vi "Elemente auswerten_Debug_Ablaufvariant.vi"(0 "GObject (Eingang)":refnum<vi>, 3 "Sprachauswahl":u16, 5 "Fehler (Eingang, kein Fehler)":errorcluster, 6 "Index":i32, 8 "ClassID":u32) -> (14 "Strings [4]":string[](array[string]), 15 "Cluster Elemente[]":refnum<vi>[](array[refnum]), 19 "error out":errorcluster)   [LabVIEW 2020, in "Sprachverwaltung.lvlib"]
uses:
  Sprachverwaltung.lvlib
  FGV Aktion Tabelle zerlegen.ctl
panel:
  # "3 Generic \n4 Decoration \n5 Text \n6 Control \n7 ColorBox \n8 Boolean \n9 RefNum \n10 Variant \n11 Path \n12 ListBox \n13 Table \n14 Array \n15 Picture \n16 ActiveXContainer \n17 Numeric \n18 Digital \n19 NamedNumeric \n20 ColorRamp \n21 Slide \n22 GraphOrChart \n23 WaveformChart \n24 WaveformGraph \n25 IntensityChart \n26 IntensityGraph \n27 String \n28 IOName \n29 ComboBox \n30 Cluster \n31 Panel \n32 Knob \n33 NumWithScale \n34 Ring \n35 Enum \n36 GObject \n37 Plot \n38 Cursor \n39 NumericText \n40 Scale \n41 ColorScale \n42 GraphScale \n43 ColorGraphScale \n44 TypedRefNum \n45 OldKnobScale \n46 MCListbox \n47 MeasureData \n48 BVTag \n49 DAQName \n50 VISAName \n51 IVIName \n52 SlideScale \n54 Page \n55 TabControl \n56 ConPane"
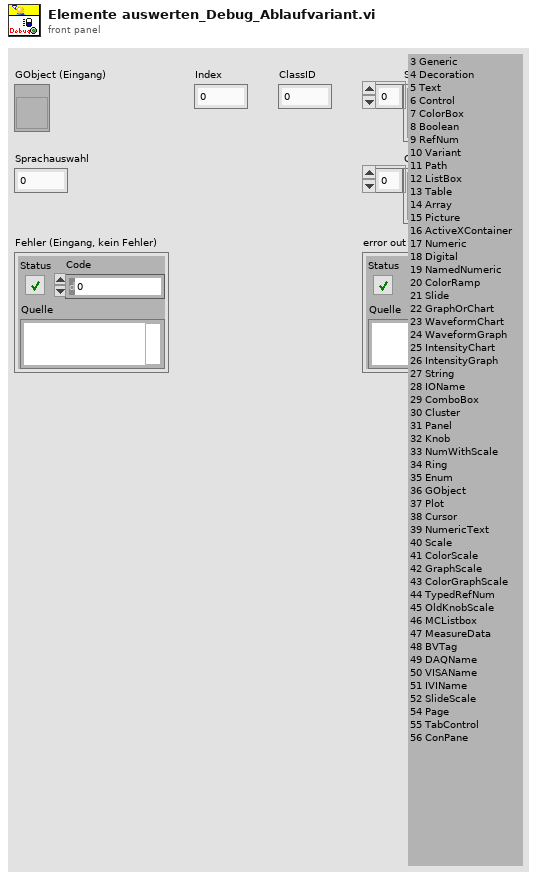
[diagram p1: front panel]
types:
  T1 = typedef "Sprachverwaltung.lvlib/FGV Aktion Tabelle zerlegen.ctl" = enum16{"laden", "vereinzeln", "speichern"}
  T2 = typedef "LVStringsAndValuesArrayTypeDef.ctl" = cluster{"String":string, "Value":ext}[]
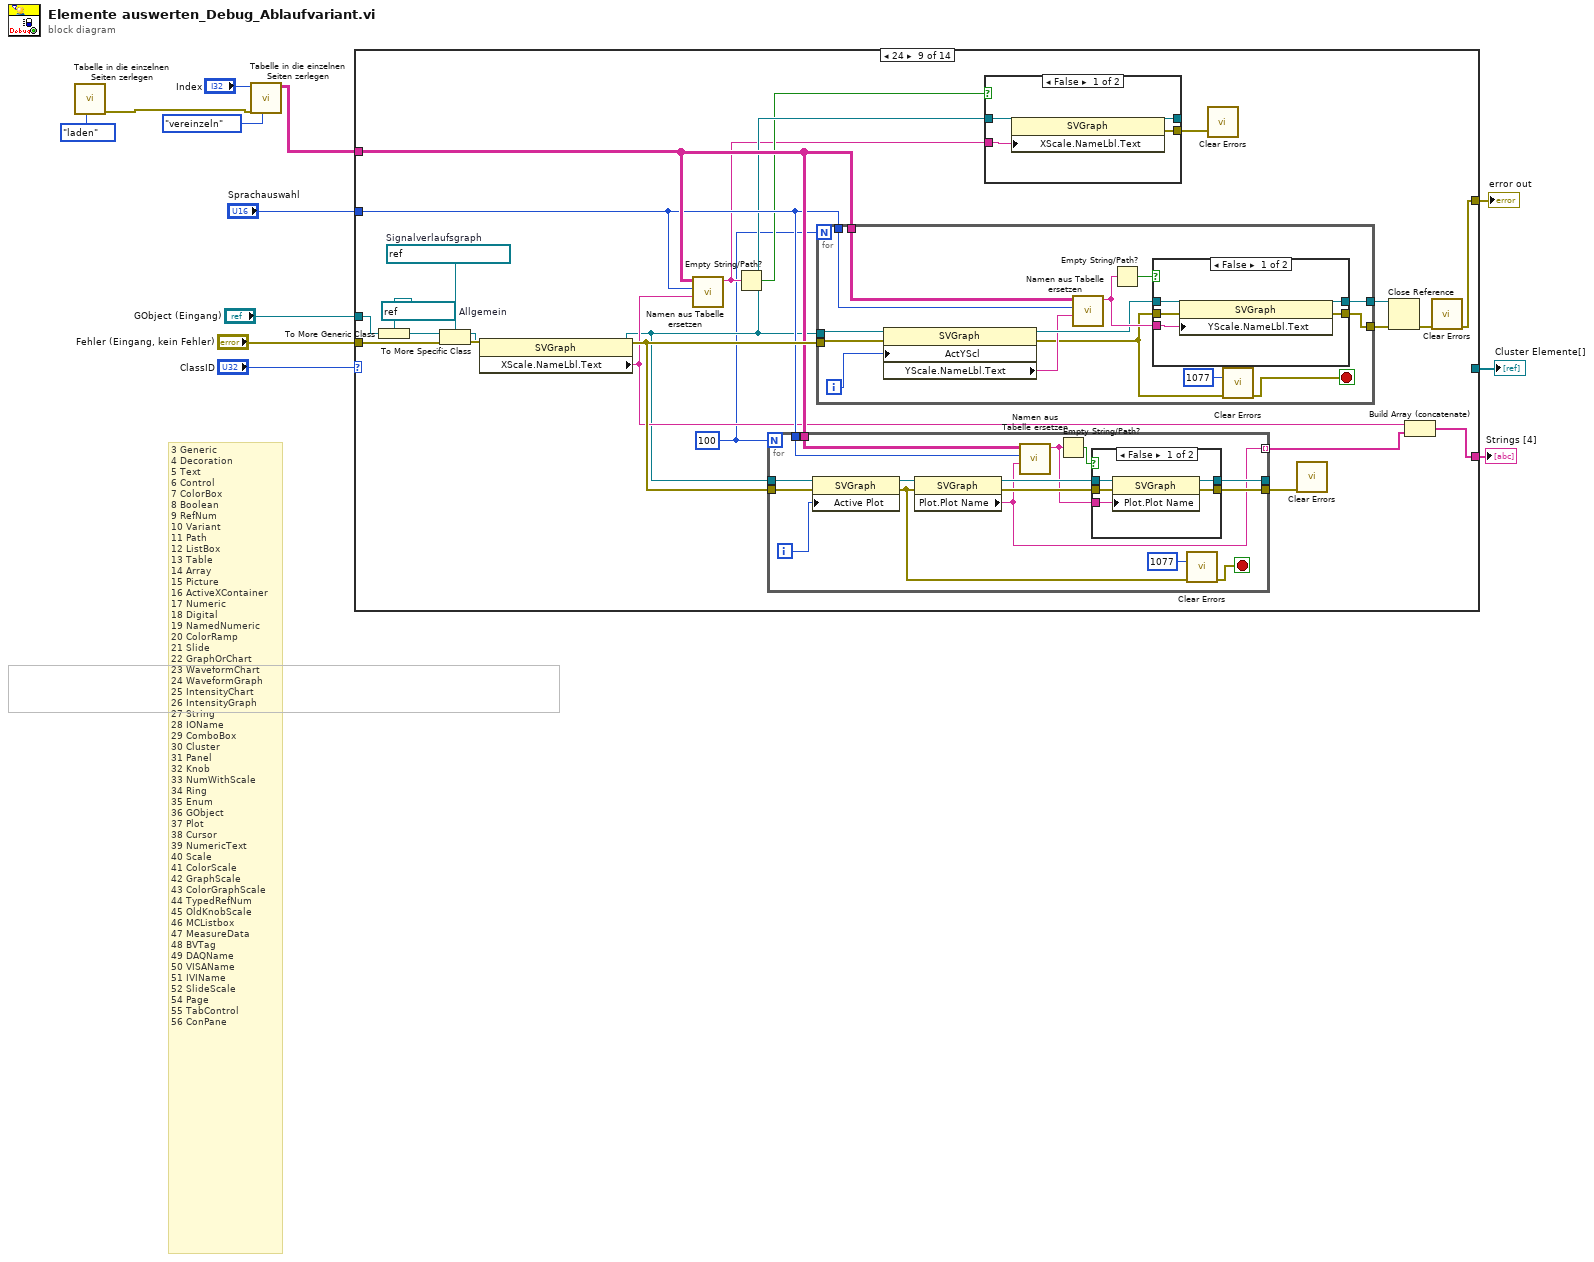
[diagram p0: block diagram]
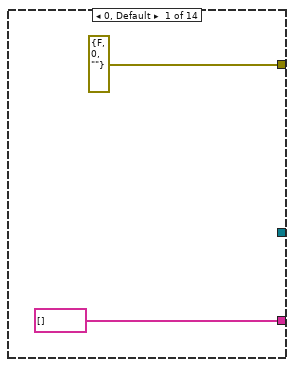
[diagram p2: hidden frame]
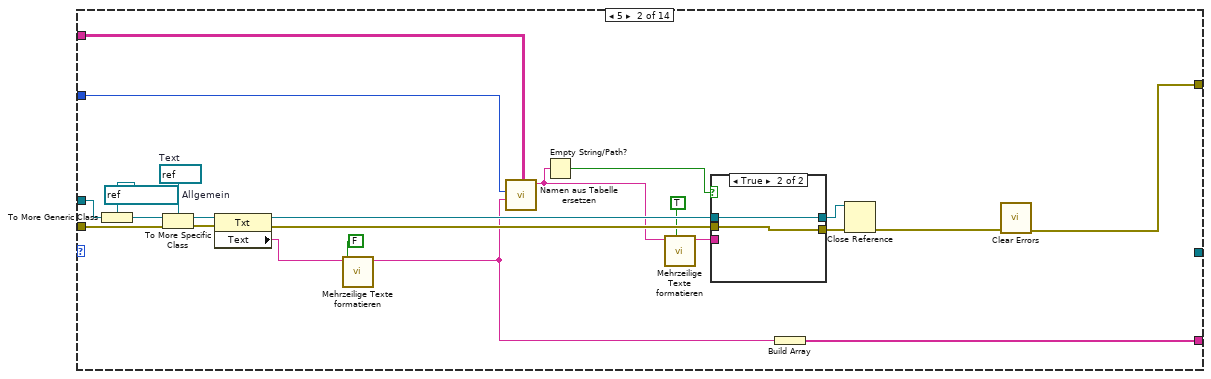
[diagram p3: hidden frame]
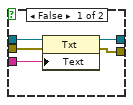
[diagram p4: hidden frame]
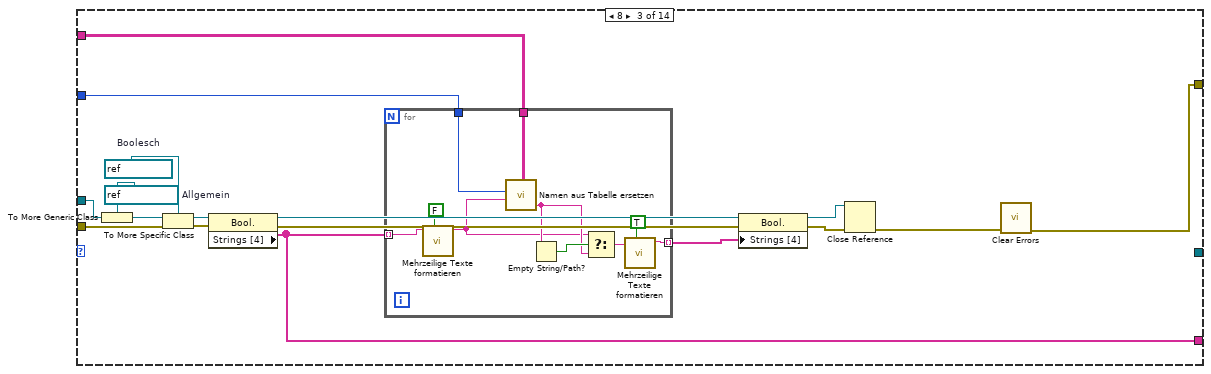
[diagram p5: hidden frame]
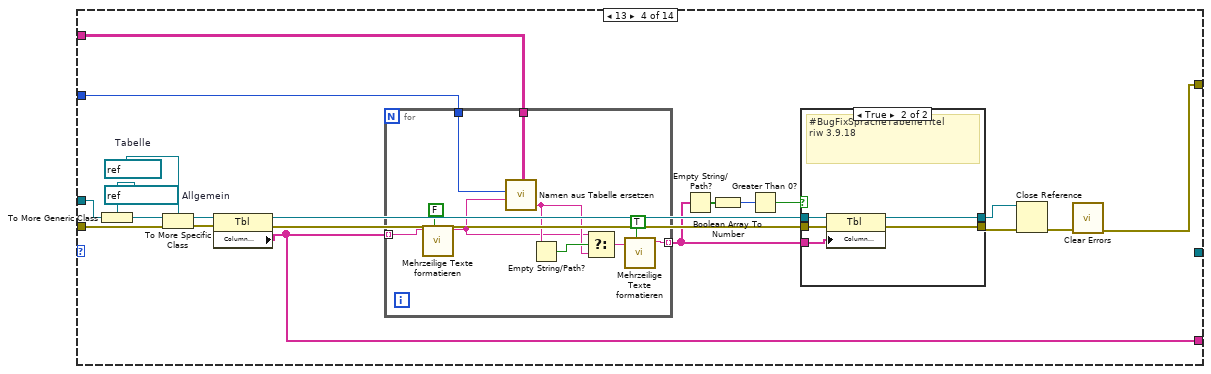
[diagram p6: hidden frame]
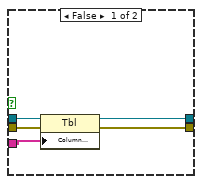
[diagram p7: hidden frame]
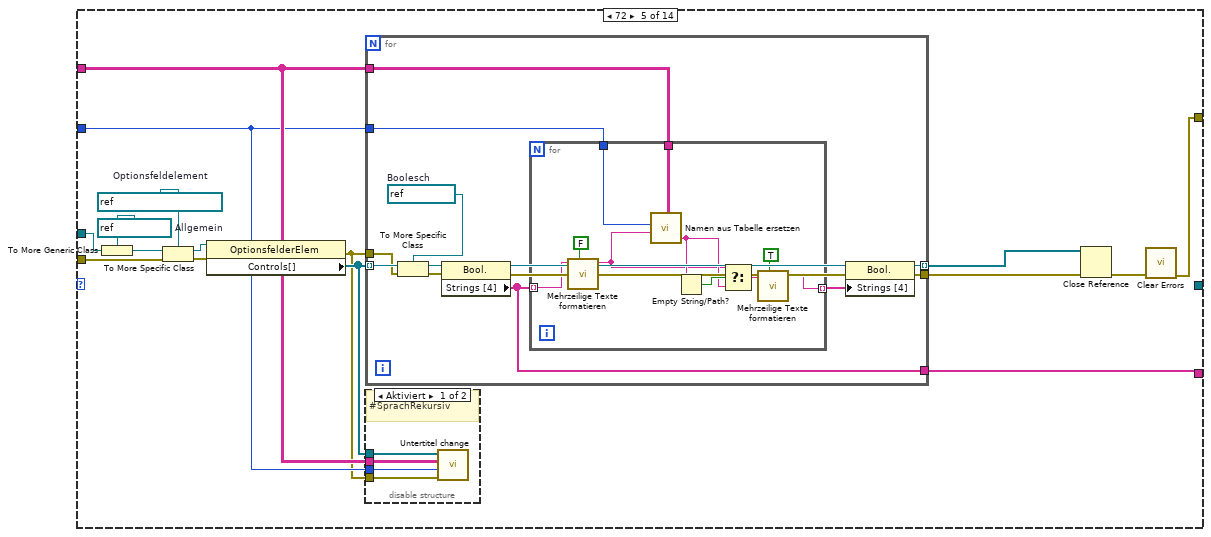
[diagram p8: hidden frame]
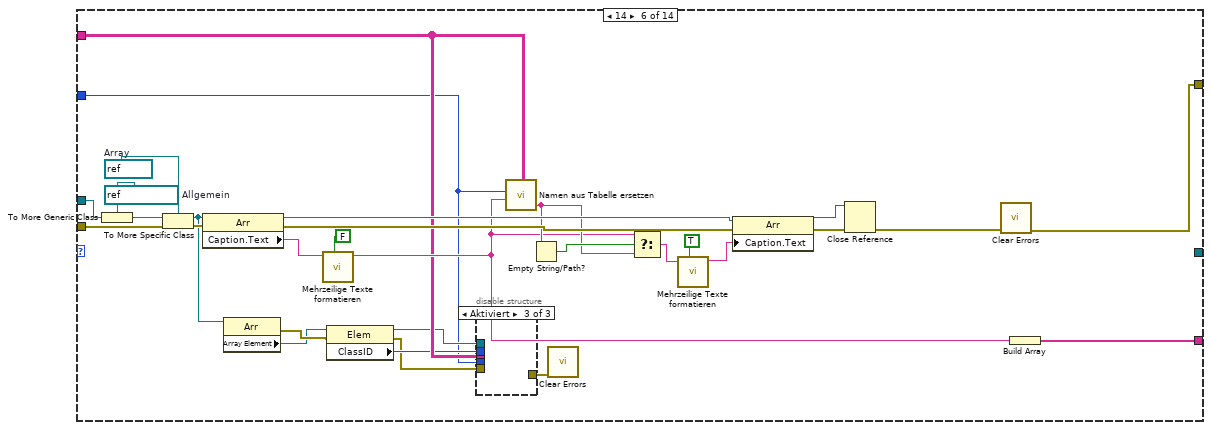
[diagram p10: hidden frame]
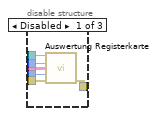
[diagram p11: hidden frame]
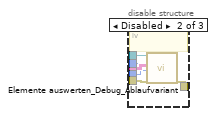
[diagram p12: hidden frame]
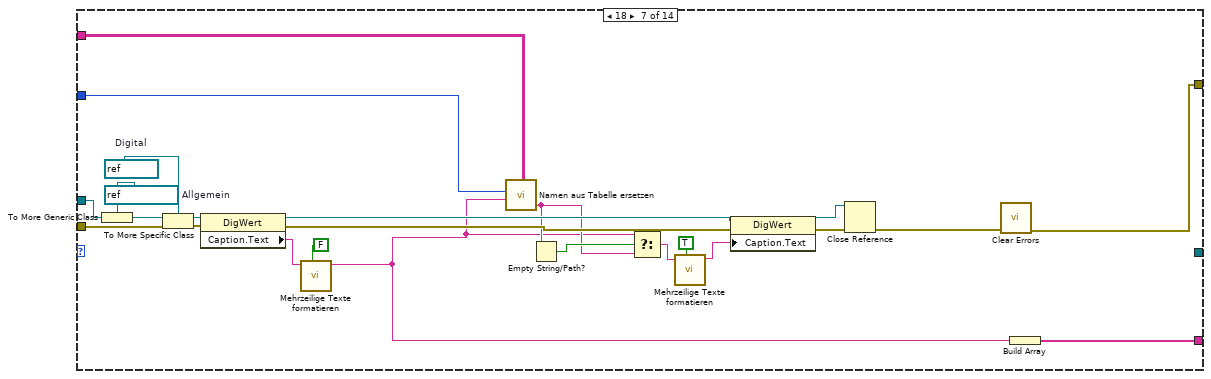
[diagram p13: hidden frame]
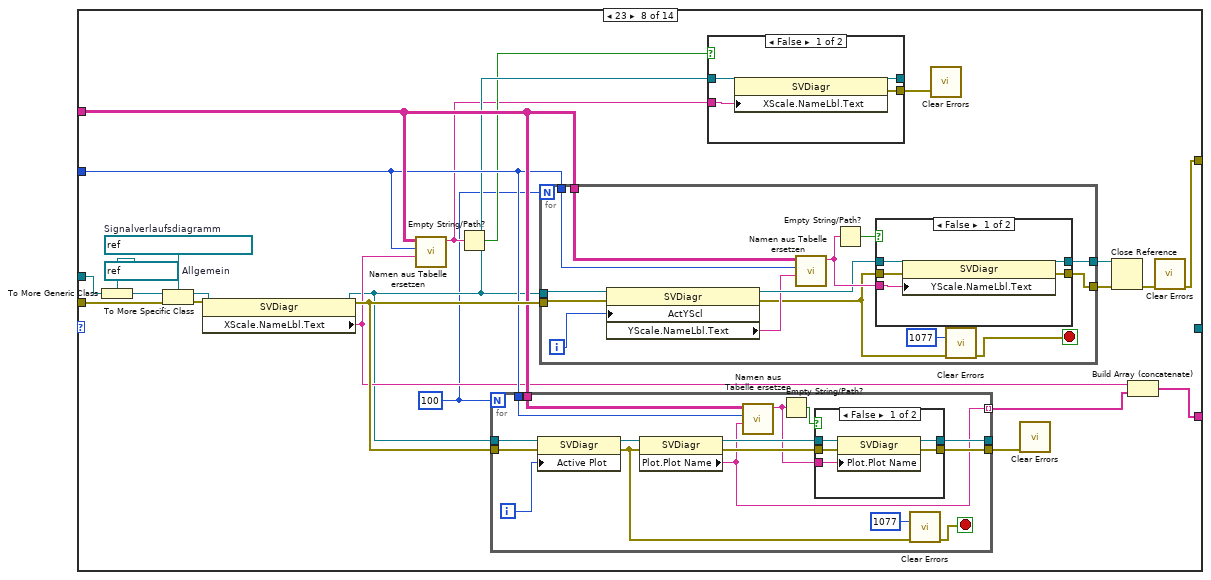
[diagram p14: hidden frame]
diagram:
  # "3 Generic \n4 Decoration \n5 Text \n6 Control \n7 ColorBox \n8 Boolean \n9 RefNum \n10 Variant \n11 Path \n12 ListBox \n13 Table \n14 Array \n15 Picture \n16 ActiveXContainer \n17 Numeric \n18 Digital \n19 NamedNumeric \n20 ColorRamp \n21 Slide \n22 GraphOrChart \n23 WaveformChart \n24 WaveformGraph \n25 IntensityChart \n26 IntensityGraph \n27 String \n28 IOName \n29 ComboBox \n30 Cluster \n31 Panel \n32 Knob \n33 NumWithScale \n34 Ring \n35 Enum \n36 GObject \n37 Plot \n38 Cursor \n39 NumericText \n40 Scale \n41 ColorScale \n42 GraphScale \n43 ColorGraphScale \n44 TypedRefNum \n45 OldKnobScale \n46 MCListbox \n47 MeasureData \n48 BVTag \n49 DAQName \n50 VISAName \n51 IVIName \n52 SlideScale \n54 Page \n55 TabControl \n56 ConPane"
  n1 = call "Tabelle in die einzelnen Seiten zerlegen.vi"("Aktion"=FGV_Aktion_Tabelle_zerlegen."laden") -> ("error out"=w1:errorcluster)  [unwired: 8 in, 2 out]
  n2 = call "Tabelle in die einzelnen Seiten zerlegen.vi"("Aktion"=FGV_Aktion_Tabelle_zerlegen."vereinzeln", "error in (no error)"=w1, "Index (Seite)"="Index") -> ("Sprachliste"=w4:string[][])  [unwired: 6 in, 2 out]
  n3 = case shown="24" "ClassID" {
    tunnel: "GObject (Eingang)" -> [_ w37 w61 w91 w127 w184 w220 w243 w315 w380 w438 w481 w509 w552]
    tunnel: "Fehler (Eingang, kein Fehler)" -> [_ w34 w58 w88 w124 w181 w217 w240 w312 w377 w435 w478 w506 w549]
    tunnel: w4 -> [_ w30 w56 w86 w114 w162 w213 w228 w302 w366 w430 w470 w494 w537]
    tunnel: "Sprachauswahl" -> [_ w23 w55 w85 w113 w157 w212 w227 w301 w365 w429 w469 w495 w536]
    tunnel: [string[] [] ("Strings [4]") w22 w48 w79 w118 w172 w205 w230 w304 w373 w420 w457 w498 w530] -> w12
    tunnel: [_ _ _ _ _ _ _ _ _ w370 _ _ _ _] -> w7
    tunnel: [errorcluster {"status"=FALSE, "code"=0, "source"=""} ("error out") w21 w47 w78 w121 w173 w206 w229 w303 w368 w419 w456 w497 w529] -> w6
    frame 0, Default {
    }
    frame 5 {
      w33 = refnum<vi> refnum  # Text
      w36 = refnum<vi> refnum  # Allgemein
      n4 = To More Generic Class(target class=w36, reference=w37) -> (generic class reference=w35:refnum<vi>)
      n5 = To More Specific Class(target class=w33, reference=w35, error in=w34) -> (specific class reference=w32:refnum<vi>, error out=w31:errorcluster)
      n6 = property class="Txt"(reference=w32, error in=w31) -> (reference out=w28:refnum<vi>, error out=w29:errorcluster, "Text"=w20:string)
      n7 = call "Mehrzeilige Texte formatieren.vi"("Zurück formatieren"=FALSE, "string"=w20) -> ("result string"=w19:string)  [unwired: 9 in]
      n8 = call "Namen aus Tabelle ersetzen.vi"("Regulärer Ausdruck"=w19, "Sprachauswahl"=w23, "Tabelle"=w30) -> ("Übersetzung"=w16:string)  [unwired: 8 in]
      n9 = Empty String/Path?(string/path=w16) -> (empty?=w24:bool)
      n10 = call "Mehrzeilige Texte formatieren.vi"("Zurück formatieren"=TRUE, "string"=w16) -> ("result string"=w15:string)  [unwired: 9 in]
      n11 = case shown="True" w24 {
        tunnel: w29 -> [w42 w43]
        tunnel: w28 -> [w41 w44]
        tunnel: w15 -> [w40 _]
        tunnel: [w39 w43] -> w27
        tunnel: [w38 w44] -> w26
        frame False {
          n12 = property class="Txt"(reference=w41, error in=w42, "Text"=w40) -> (reference out=w38:refnum<vi>, error out=w39:errorcluster)
        }
        frame True {
        }
      }
      n13 = Build Array(w19) -> (w22:string[])
      n14 = Close Reference(reference=w26, error in (no error)=w27) -> (error out=w25:errorcluster)
      n15 = call <vilib>:"Clear Errors.vi"("error in (no error)"=w25) -> ("error out"=w21:errorcluster)  [unwired: 5 in, 1 out]
    }
    frame 8 {
      w57 = refnum<vi> refnum  # Boolesch
      w60 = refnum<vi> refnum  # Allgemein
      n16 = To More Generic Class(target class=w60, reference=w61) -> (generic class reference=w59:refnum<vi>)
      n17 = To More Specific Class(target class=w57, reference=w59, error in=w58) -> (specific class reference=w45:refnum<vi>, error out=w46:errorcluster)
      n18 = property class="Bool."(reference=w45, error in=w46) -> (reference out=w53:refnum<vi>, error out=w54:errorcluster, "Strings [4]"=w48:string[])
      n19 = for {
        tunnel: w48 -> [w66] mode=indexing
        tunnel: w56 -> [w71]
        tunnel: w55 -> [w70]
        tunnel: [w62] -> w49 mode=indexing
        n20 = call "Mehrzeilige Texte formatieren.vi"("Zurück formatieren"=FALSE, "string"=w66) -> ("result string"=w65:string)  [unwired: 9 in]
        n21 = call "Namen aus Tabelle ersetzen.vi"("Regulärer Ausdruck"=w65, "Sprachauswahl"=w70, "Tabelle"=w71) -> ("Übersetzung"=w68:string)  [unwired: 8 in]
        n22 = Empty String/Path?(string/path=w68) -> (empty?=w69:bool)
        n23 = Select(t=w65, s=w69, f=w68) -> (s? t:f=w63:string)
        n24 = call "Mehrzeilige Texte formatieren.vi"("Zurück formatieren"=TRUE, "string"=w63) -> ("result string"=w62:string)  [unwired: 9 in]
      }
      n25 = property class="Bool."(reference=w53, error in=w54, "Strings [4]"=w49) -> (reference out=w51:refnum<vi>, error out=w52:errorcluster)
      n26 = Close Reference(reference=w51, error in (no error)=w52) -> (error out=w50:errorcluster)
      n27 = call <vilib>:"Clear Errors.vi"("error in (no error)"=w50) -> ("error out"=w47:errorcluster)  [unwired: 5 in, 1 out]
    }
    frame 13 {
      w87 = refnum<vi> refnum  # Tabelle
      w90 = refnum<vi> refnum  # Allgemein
      n28 = To More Generic Class(target class=w90, reference=w91) -> (generic class reference=w89:refnum<vi>)
      n29 = To More Specific Class(target class=w87, reference=w89, error in=w88) -> (specific class reference=w76:refnum<vi>, error out=w77:errorcluster)
      n30 = property class="Tbl"(reference=w76, error in=w77) -> (reference out=w83:refnum<vi>, error out=w84:errorcluster, "Column Headers[]"=w79:string[])
      n31 = for {
        tunnel: w79 -> [w106] mode=indexing
        tunnel: w86 -> [w111]
        tunnel: w85 -> [w110]
        tunnel: [w102] -> w75 mode=indexing
        n32 = call "Mehrzeilige Texte formatieren.vi"("Zurück formatieren"=FALSE, "string"=w106) -> ("result string"=w105:string)  [unwired: 9 in]
        n33 = call "Namen aus Tabelle ersetzen.vi"("Regulärer Ausdruck"=w105, "Sprachauswahl"=w110, "Tabelle"=w111) -> ("Übersetzung"=w108:string)  [unwired: 8 in]
        n34 = Empty String/Path?(string/path=w108) -> (empty?=w109:bool)
        n35 = Select(t=w105, s=w109, f=w108) -> (s? t:f=w103:string)
        n36 = call "Mehrzeilige Texte formatieren.vi"("Zurück formatieren"=TRUE, "string"=w103) -> ("result string"=w102:string)  [unwired: 9 in]
      }
      n37 = Empty String/Path?(string/path=w75) -> (empty?=w74:bool[])
      n38 = Boolean Array To Number(Boolean array=w74) -> (number=w73:u32)
      n39 = Greater Than 0?(x=w73) -> (x > 0?=w72:bool)
      n40 = case shown="True" w72 {
        tunnel: w84 -> [w96 w99]
        tunnel: w83 -> [w95 w101]
        tunnel: [w94 w98] -> w82
        tunnel: [w93 w100] -> w81
        tunnel: w75 -> [w92 w97]
        frame False {
          n41 = property class="Tbl"(reference=w95, error in=w96, "Column Headers[]"=w92) -> (reference out=w93:refnum<vi>, error out=w94:errorcluster)
        }
        frame True {
          # "#BugFixSpracheTabelleTitel\nriw 3.9.18"
          n42 = property class="Tbl"(reference=w101, error in=w99, "Column Headers[]"=w97) -> (reference out=w100:refnum<vi>, error out=w98:errorcluster)
        }
      }
      n43 = Close Reference(reference=w81, error in (no error)=w82) -> (error out=w80:errorcluster)
      n44 = call <vilib>:"Clear Errors.vi"("error in (no error)"=w80) -> ("error out"=w78:errorcluster)  [unwired: 5 in, 1 out]
    }
    frame 72 {
      w123 = refnum<vi> refnum  # Optionsfeldelement
      w126 = refnum<vi> refnum  # Allgemein
      n45 = To More Generic Class(target class=w126, reference=w127) -> (generic class reference=w125:refnum<vi>)
      n46 = To More Specific Class(target class=w123, reference=w125, error in=w124) -> (specific class reference=w119:refnum<vi>, error out=w120:errorcluster)
      n47 = property class="OptionsfelderElem"(reference=w119, error in=w120) -> (error out=w112:errorcluster, "Controls[]"=w115:refnum<vi>[])  [unwired: 1 out]
      n48 = for {
        tunnel: w114 -> [w134]
        tunnel: w113 -> [w133]
        tunnel: w115 -> [w135] mode=indexing
        tunnel: [w142] -> w118
        tunnel: w112 -> [w132]
        tunnel: [w137] -> w117
        tunnel: [w136] -> w116 mode=indexing
        w144 = refnum<vi> refnum  # Boolesch
        n49 = To More Specific Class(target class=w144, reference=w135, error in=w132) -> (specific class reference=w143:refnum<vi>, error out=w141:errorcluster)
        n50 = property class="Bool."(reference=w143, error in=w141) -> (reference out=w140:refnum<vi>, error out=w139:errorcluster, "Strings [4]"=w142:string[])
        n51 = for {
          tunnel: w134 -> [w154]
          tunnel: w133 -> [w153]
          tunnel: [w146] -> w138 mode=indexing
          tunnel: w142 -> [w145] mode=indexing
          n52 = call "Mehrzeilige Texte formatieren.vi"("Zurück formatieren"=FALSE, "string"=w145) -> ("result string"=w149:string)  [unwired: 9 in]
          n53 = call "Namen aus Tabelle ersetzen.vi"("Regulärer Ausdruck"=w149, "Sprachauswahl"=w153, "Tabelle"=w154) -> ("Übersetzung"=w151:string)  [unwired: 8 in]
          n54 = Empty String/Path?(string/path=w151) -> (empty?=w152:bool)
          n55 = Select(t=w149, s=w152, f=w151) -> (s? t:f=w147:string)
          n56 = call "Mehrzeilige Texte formatieren.vi"("Zurück formatieren"=TRUE, "string"=w147) -> ("result string"=w146:string)  [unwired: 9 in]
        }
        n57 = property class="Bool."(reference=w140, error in=w139, "Strings [4]"=w138) -> (reference out=w136:refnum<vi>, error out=w137:errorcluster)
      }
      n58 = disable-structure shown="Aktiviert" {
        disable-tunnel: w115 -> [w131 _]
        disable-tunnel: w114 -> [w130 _]
        disable-tunnel: w113 -> [w129 _]
        disable-tunnel: w112 -> [w128 _]
        frame Enabled {
          # "#SprachRekursiv"
          n59 = call "Untertitel change.vi"("Fehler (Eingang, kein Fehler)"=w128, "Sprachauswahl"=w129, "Sprachdatei"=w130, "Controls[]"=w131) -> ()  [unwired: 7 in, 1 out]
        }
        frame Disabled {
        }
      }
      n60 = Close Reference(reference=w116, error in (no error)=w117) -> (error out=w122:errorcluster)
      n61 = call <vilib>:"Clear Errors.vi"("error in (no error)"=w122) -> ("error out"=w121:errorcluster)  [unwired: 5 in, 1 out]
    }
    frame 14 {
      w180 = refnum<vi> refnum  # Array
      w183 = refnum<vi> refnum  # Allgemein
      n62 = To More Generic Class(target class=w183, reference=w184) -> (generic class reference=w182:refnum<vi>)
      n63 = To More Specific Class(target class=w180, reference=w182, error in=w181) -> (specific class reference=w163:refnum<vi>, error out=w179:errorcluster)
      n64 = property class="Arr"(reference=w163, error in=w179) -> (reference out=w177:refnum<vi>, error out=w178:errorcluster, "Caption.Text"=w168:string)
      n65 = property class="Arr"(reference=w163) -> (error out=w161:errorcluster, "Array Element"=w160:refnum<vi>)  [unwired: 1 in, 1 out]
      n66 = call "Mehrzeilige Texte formatieren.vi"("Zurück formatieren"=FALSE, "string"=w168) -> ("result string"=w167:string)  [unwired: 9 in]
      n67 = property class="Elem"(reference=w160, error in=w161) -> (reference out=w158:refnum<vi>, error out=w156:errorcluster, "ClassID"=w159:u32)
      n68 = disable-structure shown="Aktiviert" {
        disable-tunnel: w162 -> [w190 w196 _]
        disable-tunnel: w159 -> [w189 w195 _]
        disable-tunnel: w158 -> [w188 w194 _]
        disable-tunnel: w157 -> [w187 w193 _]
        disable-tunnel: w156 -> [w186 w192 _]
        disable-tunnel: [w185 w191 _] -> w155
        frame Disabled {
          n69 = call "Auswertung Registerkarte.vi"("GObject (Eingang)"=w188, "ClassID"=w189, "all rows"=w190, "Sprachauswahl"=w187, "Fehler (Eingang, kein Fehler)"=w186) -> ("error out"=w185:errorcluster)  [unwired: 9 in, 1 out]
        }
        frame Disabled {
          # "#SprachRekursiv"
          n70 = call "Elemente auswerten_Debug_Ablaufvariant.vi"("GObject (Eingang)"=w194, 2:w196, "Sprachauswahl"=w193, "Fehler (Eingang, kein Fehler)"=w192, "ClassID"=w195) -> ("error out"=w191:errorcluster)  [unwired: 12 in, 2 out]
        }
        frame Enabled {
        }
      }
      n71 = call "Namen aus Tabelle ersetzen.vi"("Regulärer Ausdruck"=w167, "Sprachauswahl"=w157, "Tabelle"=w162) -> ("Übersetzung"=w170:string)  [unwired: 8 in]
      n72 = Empty String/Path?(string/path=w170) -> (empty?=w171:bool)
      n73 = call <vilib>:"Clear Errors.vi"("error in (no error)"=w155) -> ()  [unwired: 5 in, 2 out]
      n74 = Select(t=w167, s=w171, f=w170) -> (s? t:f=w165:string)
      n75 = call "Mehrzeilige Texte formatieren.vi"("Zurück formatieren"=TRUE, "string"=w165) -> ("result string"=w164:string)  [unwired: 9 in]
      n76 = property class="Arr"(reference=w177, error in=w178, "Caption.Text"=w164) -> (reference out=w175:refnum<vi>, error out=w176:errorcluster)
      n77 = Close Reference(reference=w175, error in (no error)=w176) -> (error out=w174:errorcluster)
      n78 = call <vilib>:"Clear Errors.vi"("error in (no error)"=w174) -> ("error out"=w173:errorcluster)  [unwired: 5 in, 1 out]
      n79 = Build Array(w167) -> (w172:string[])
    }
    frame 18 {
      w216 = refnum<vi> refnum  # Digital
      w219 = refnum<vi> refnum  # Allgemein
      n80 = To More Generic Class(target class=w219, reference=w220) -> (generic class reference=w218:refnum<vi>)
      n81 = To More Specific Class(target class=w216, reference=w218, error in=w217) -> (specific class reference=w215:refnum<vi>, error out=w214:errorcluster)
      n82 = property class="DigWert"(reference=w215, error in=w214) -> (reference out=w210:refnum<vi>, error out=w211:errorcluster, "Caption.Text"=w201:string)
      n83 = call "Mehrzeilige Texte formatieren.vi"("Zurück formatieren"=FALSE, "string"=w201) -> ("result string"=w200:string)  [unwired: 9 in]
      n84 = call "Namen aus Tabelle ersetzen.vi"("Regulärer Ausdruck"=w200, "Sprachauswahl"=w212, "Tabelle"=w213) -> ("Übersetzung"=w203:string)  [unwired: 8 in]
      n85 = Empty String/Path?(string/path=w203) -> (empty?=w204:bool)
      n86 = Select(t=w200, s=w204, f=w203) -> (s? t:f=w198:string)
      n87 = call "Mehrzeilige Texte formatieren.vi"("Zurück formatieren"=TRUE, "string"=w198) -> ("result string"=w197:string)  [unwired: 9 in]
      n88 = property class="DigWert"(reference=w210, error in=w211, "Caption.Text"=w197) -> (reference out=w208:refnum<vi>, error out=w209:errorcluster)
      n89 = Close Reference(reference=w208, error in (no error)=w209) -> (error out=w207:errorcluster)
      n90 = call <vilib>:"Clear Errors.vi"("error in (no error)"=w207) -> ("error out"=w206:errorcluster)  [unwired: 5 in, 1 out]
      n91 = Build Array(w200) -> (w205:string[])
    }
    frame 23 {
      w221 = 100
      w239 = refnum<vi> refnum  # Signalverlaufsdiagramm
      w242 = refnum<vi> refnum  # Allgemein
      n92 = To More Generic Class(target class=w242, reference=w243) -> (generic class reference=w241:refnum<vi>)
      n93 = To More Specific Class(target class=w239, reference=w241, error in=w240) -> (specific class reference=w238:refnum<vi>, error out=w237:errorcluster)
      n94 = property class="SVDiagr"(reference=w238, error in=w237) -> (reference out=w225:refnum<vi>, error out=w235:errorcluster, "XScale.NameLbl.Text"=w226:string)
      n95 = call "Namen aus Tabelle ersetzen.vi"("Regulärer Ausdruck"=w226, "Sprachauswahl"=w227, "Tabelle"=w228) -> ("Übersetzung"=w223:string)  [unwired: 8 in]
      n96 = Empty String/Path?(string/path=w223) -> (empty?=w224:bool)
      n97 = for {
        N: w221 -> [_]
        tunnel: w225 -> [w264]
        tunnel: w235 -> [w261]
        tunnel: w228 -> [w260]
        tunnel: w227 -> [w259]
        tunnel: [w255] -> _
        tunnel: [w254] -> w232
        tunnel: [w252] -> w231 mode=indexing
        i -> [w263]
        stop <- w250 stop-if-true
        n98 = property class="SVDiagr"(reference=w264, error in=w261, "Active Plot"=w263) -> (reference out=w262:refnum<vi>, error out=w249:errorcluster)
        n99 = property class="SVDiagr"(reference=w262, error in=w249) -> (reference out=w258:refnum<vi>, error out=w257:errorcluster, "Plot.Plot Name"=w252:string)
        n100 = call "Namen aus Tabelle ersetzen.vi"("Regulärer Ausdruck"=w252, "Sprachauswahl"=w259, "Tabelle"=w260) -> ("Übersetzung"=w253:string)  [unwired: 8 in]
        n101 = Empty String/Path?(string/path=w253) -> (empty?=w256:bool)
        n102 = case shown="False" w256 {
          tunnel: w258 -> [w269 w271]
          tunnel: w257 -> [w268 w270]
          tunnel: [w267 w271] -> w255
          tunnel: [w266 w270] -> w254
          tunnel: w253 -> [w265 _]
          frame False {
            n103 = property class="SVDiagr"(reference=w269, error in=w268, "Plot.Plot Name"=w265) -> (reference out=w267:refnum<vi>, error out=w266:errorcluster)
          }
          frame True {
          }
        }
        n104 = call <vilib>:"Clear Errors.vi"("error in (no error)"=w249, "specific error code to clear (0: all)"=1077) -> ("error out"=w250:errorcluster)  [unwired: 4 in, 1 out]
      }
      n105 = for {
        N: w221 -> [_]
        tunnel: w228 -> [w285]
        tunnel: w227 -> [w280]
        tunnel: w225 -> [w278]
        tunnel: w235 -> [w279]
        tunnel: [w282] -> w234
        tunnel: [w281] -> w233
        i -> [w276]
        stop <- w274 stop-if-true
        n106 = property class="SVDiagr"(reference=w278, error in=w279, "ActYScl"=w276) -> (reference out=w277:refnum<vi>, error out=w273:errorcluster, "YScale.NameLbl.Text"=w275:string)
        n107 = call "Namen aus Tabelle ersetzen.vi"("Regulärer Ausdruck"=w275, "Sprachauswahl"=w280, "Tabelle"=w285) -> ("Übersetzung"=w283:string)  [unwired: 8 in]
        n108 = Empty String/Path?(string/path=w283) -> (empty?=w284:bool)
        n109 = case shown="False" w284 {
          tunnel: w273 -> [w290 w291]
          tunnel: w277 -> [w289 w292]
          tunnel: [w288 w291] -> w281
          tunnel: [w287 w292] -> w282
          tunnel: w283 -> [w286 _]
          frame False {
            n110 = property class="SVDiagr"(reference=w289, error in=w290, "YScale.NameLbl.Text"=w286) -> (reference out=w287:refnum<vi>, error out=w288:errorcluster)
          }
          frame True {
          }
        }
        n111 = call <vilib>:"Clear Errors.vi"("error in (no error)"=w273, "specific error code to clear (0: all)"=1077) -> ("error out"=w274:errorcluster)  [unwired: 4 in, 1 out]
      }
      n112 = case shown="False" w224 {
        tunnel: w225 -> [w247 w248]
        tunnel: [w246 _] -> w222
        tunnel: [w245 w248] -> _
        tunnel: w223 -> [w244 _]
        frame False {
          n113 = property class="SVDiagr"(reference=w247, "XScale.NameLbl.Text"=w244) -> (reference out=w245:refnum<vi>, error out=w246:errorcluster)  [unwired: 1 in]
        }
        frame True {
        }
      }
      n114 = call <vilib>:"Clear Errors.vi"("error in (no error)"=w222) -> ()  [unwired: 5 in, 2 out]
      n115 = call <vilib>:"Clear Errors.vi"("error in (no error)"=w232) -> ()  [unwired: 5 in, 2 out]
      n116 = Close Reference(reference=w234, error in (no error)=w233) -> (error out=w236:errorcluster)
      n117 = Build Array (concatenate)(w226, w231) -> (w230:string[])
      n118 = call <vilib>:"Clear Errors.vi"("error in (no error)"=w236) -> ("error out"=w229:errorcluster)  [unwired: 5 in, 1 out]
    }
    frame 24 {
      w294 = refnum<vi> refnum  # Signalverlaufsgraph
      w295 = 100
      w314 = refnum<vi> refnum  # Allgemein
      n119 = To More Generic Class(target class=w314, reference=w315) -> (generic class reference=w313:refnum<vi>)
      n120 = To More Specific Class(target class=w294, reference=w313, error in=w312) -> (specific class reference=w293:refnum<vi>, error out=w311:errorcluster)
      n121 = property class="SVGraph"(reference=w293, error in=w311) -> (reference out=w299:refnum<vi>, error out=w309:errorcluster, "XScale.NameLbl.Text"=w300:string)
      n122 = call "Namen aus Tabelle ersetzen.vi"("Regulärer Ausdruck"=w300, "Sprachauswahl"=w301, "Tabelle"=w302) -> ("Übersetzung"=w297:string)  [unwired: 8 in]
      n123 = Empty String/Path?(string/path=w297) -> (empty?=w298:bool)
      n124 = for {
        N: w295 -> [_]
        tunnel: w299 -> [w336]
        tunnel: w309 -> [w333]
        tunnel: w302 -> [w332]
        tunnel: w301 -> [w331]
        tunnel: [w327] -> _
        tunnel: [w326] -> w306
        tunnel: [w324] -> w305 mode=indexing
        i -> [w335]
        stop <- w322 stop-if-true
        n125 = property class="SVGraph"(reference=w336, error in=w333, "Active Plot"=w335) -> (reference out=w334:refnum<vi>, error out=w321:errorcluster)
        n126 = property class="SVGraph"(reference=w334, error in=w321) -> (reference out=w330:refnum<vi>, error out=w329:errorcluster, "Plot.Plot Name"=w324:string)
        n127 = call "Namen aus Tabelle ersetzen.vi"("Regulärer Ausdruck"=w324, "Sprachauswahl"=w331, "Tabelle"=w332) -> ("Übersetzung"=w325:string)  [unwired: 8 in]
        n128 = Empty String/Path?(string/path=w325) -> (empty?=w328:bool)
        n129 = case shown="False" w328 {
          tunnel: w330 -> [w341 w343]
          tunnel: w329 -> [w340 w342]
          tunnel: [w339 w343] -> w327
          tunnel: [w338 w342] -> w326
          tunnel: w325 -> [w337 _]
          frame False {
            n130 = property class="SVGraph"(reference=w341, error in=w340, "Plot.Plot Name"=w337) -> (reference out=w339:refnum<vi>, error out=w338:errorcluster)
          }
          frame True {
          }
        }
        n131 = call <vilib>:"Clear Errors.vi"("error in (no error)"=w321, "specific error code to clear (0: all)"=1077) -> ("error out"=w322:errorcluster)  [unwired: 4 in, 1 out]
      }
      n132 = for {
        N: w295 -> [_]
        tunnel: w302 -> [w357]
        tunnel: w301 -> [w352]
        tunnel: w299 -> [w350]
        tunnel: w309 -> [w351]
        tunnel: [w354] -> w308
        tunnel: [w353] -> w307
        i -> [w348]
        stop <- w346 stop-if-true
        n133 = property class="SVGraph"(reference=w350, error in=w351, "ActYScl"=w348) -> (reference out=w349:refnum<vi>, error out=w345:errorcluster, "YScale.NameLbl.Text"=w347:string)
        n134 = call "Namen aus Tabelle ersetzen.vi"("Regulärer Ausdruck"=w347, "Sprachauswahl"=w352, "Tabelle"=w357) -> ("Übersetzung"=w355:string)  [unwired: 8 in]
        n135 = Empty String/Path?(string/path=w355) -> (empty?=w356:bool)
        n136 = case shown="False" w356 {
          tunnel: w345 -> [w362 w363]
          tunnel: w349 -> [w361 w364]
          tunnel: [w360 w363] -> w353
          tunnel: [w359 w364] -> w354
          tunnel: w355 -> [w358 _]
          frame False {
            n137 = property class="SVGraph"(reference=w361, error in=w362, "YScale.NameLbl.Text"=w358) -> (reference out=w359:refnum<vi>, error out=w360:errorcluster)
          }
          frame True {
          }
        }
        n138 = call <vilib>:"Clear Errors.vi"("error in (no error)"=w345, "specific error code to clear (0: all)"=1077) -> ("error out"=w346:errorcluster)  [unwired: 4 in, 1 out]
      }
      n139 = case shown="False" w298 {
        tunnel: w299 -> [w319 w320]
        tunnel: [w318 _] -> w296
        tunnel: [w317 w320] -> _
        tunnel: w297 -> [w316 _]
        frame False {
          n140 = property class="SVGraph"(reference=w319, "XScale.NameLbl.Text"=w316) -> (reference out=w317:refnum<vi>, error out=w318:errorcluster)  [unwired: 1 in]
        }
        frame True {
        }
      }
      n141 = call <vilib>:"Clear Errors.vi"("error in (no error)"=w296) -> ()  [unwired: 5 in, 2 out]
      n142 = call <vilib>:"Clear Errors.vi"("error in (no error)"=w306) -> ()  [unwired: 5 in, 2 out]
      n143 = Close Reference(reference=w308, error in (no error)=w307) -> (error out=w310:errorcluster)
      n144 = Build Array (concatenate)(w300, w305) -> (w304:string[])
      n145 = call <vilib>:"Clear Errors.vi"("error in (no error)"=w310) -> ("error out"=w303:errorcluster)  [unwired: 5 in, 1 out]
    }
    frame 30 {
      w376 = refnum<vi> refnum  # Cluster
      w379 = refnum<vi> refnum  # Allgemein
      # "Eventuell die komplette Casestruktur mit allen funktionen einbauen?!!"
      n146 = To More Generic Class(target class=w379, reference=w380) -> (generic class reference=w378:refnum<vi>)
      n147 = To More Specific Class(target class=w376, reference=w378, error in=w377) -> (specific class reference=w375:refnum<vi>, error out=w374:errorcluster)
      n148 = property class="Cluster"(reference=w375, error in=w374) -> (reference out=w372:refnum<vi>, error out=w371:errorcluster, "Controls[]"=w370:refnum<vi>[], "AllObjs[]"=w367:refnum<vi>[])
      n149 = disable-structure shown="Deaktiviert" {
        disable-tunnel: w367 -> [w383 _]
        disable-tunnel: w366 -> [w382 _]
        disable-tunnel: w365 -> [w381 _]
        frame Disabled {
          n150 = for {
            tunnel: w383 -> [w389] mode=indexing
            tunnel: w382 -> [w384]
            tunnel: w381 -> [w386]
            n151 = property class="GObj"(reference=w389) -> ("ClassID"=w388:u32)  [unwired: 1 in, 2 out]
            n152 = call "Elemente auswerten_Debug_Ablaufvariant.vi"("GObject (Eingang)"=w389, 2:w384, "Sprachauswahl"=w386, "ClassID"=w388) -> ("Cluster Elemente[]"=w387:refnum<vi>[], "error out"=w385:errorcluster)  [unwired: 13 in, 1 out]
            n153 = for {
              tunnel: w384 -> [w395]
              tunnel: w385 -> [w394]
              tunnel: w386 -> [w393]
              tunnel: w387 -> [w392] mode=indexing
              n154 = property class="Elem"(reference=w392) -> (reference out=w391:refnum<vi>, "ClassID"=w390:u32)  [unwired: 1 in, 1 out]
              n155 = call "Elemente auswerten_Debug_Ablaufvariant.vi"("GObject (Eingang)"=w391, 2:w395, "Sprachauswahl"=w393, "Fehler (Eingang, kein Fehler)"=w394, "ClassID"=w390) -> ()  [unwired: 12 in, 3 out]
            }
          }
        }
        frame Enabled {
        }
      }
      n156 = for {
        tunnel: w366 -> [w396]
        tunnel: w371 -> [w400]
        tunnel: w372 -> [_]
        tunnel: w365 -> [w398]
        tunnel: w370 -> [w397] mode=indexing
        tunnel: [w403] -> w373 mode=indexing
        tunnel: [w407] -> w369
        n157 = property class="Elem"(reference=w397, error in=w400) -> (reference out=w408:refnum<vi>, error out=w399:errorcluster, "Caption.Text"=w404:string)
        n158 = call "Mehrzeilige Texte formatieren.vi"("Zurück formatieren"=FALSE, "string"=w404) -> ("result string"=w403:string)  [unwired: 9 in]
        n159 = call "Namen aus Tabelle ersetzen.vi"("Regulärer Ausdruck"=w403, "Sprachauswahl"=w398, "Tabelle"=w396) -> ("Übersetzung"=w402:string)  [unwired: 8 in]
        n160 = Empty String/Path?(string/path=w402) -> (empty?=w409:bool)
        n161 = call "Mehrzeilige Texte formatieren.vi"("Zurück formatieren"=TRUE, "string"=w402) -> ("result string"=w401:string)  [unwired: 9 in]
        n162 = case shown="True" w409 {
          tunnel: w399 -> [w416 w417]
          tunnel: w408 -> [w415 w418]
          tunnel: w401 -> [w414 _]
          tunnel: [w413 w417] -> w411
          tunnel: [w412 w418] -> w410
          frame False {
            n163 = property class="Elem"(reference=w415, error in=w416, "Caption.Text"=w414) -> (reference out=w412:refnum<vi>, error out=w413:errorcluster)
          }
          frame True {
          }
        }
        n164 = Close Reference(reference=w410, error in (no error)=w411) -> (error out=w407:errorcluster)
      }
      n165 = call <vilib>:"Clear Errors.vi"("error in (no error)"=w369) -> ("error out"=w368:errorcluster)  [unwired: 5 in, 1 out]
    }
    frame 34 {
      w434 = refnum<vi> refnum  # Ring
      w437 = refnum<vi> refnum  # Allgemein
      n166 = To More Generic Class(target class=w437, reference=w438) -> (generic class reference=w436:refnum<vi>)
      n167 = To More Specific Class(target class=w434, reference=w436, error in=w435) -> (specific class reference=w433:refnum<vi>, error out=w432:errorcluster)
      n168 = property class="Ring"(reference=w433, error in=w432) -> (reference out=w427:refnum<vi>, error out=w428:errorcluster, "StringsAndValues[]"=w431:T2)
      n169 = for {
        tunnel: w431 -> [w450] mode=indexing
        tunnel: w430 -> [w455]
        tunnel: w429 -> [w447]
        tunnel: [w448] -> w423 mode=indexing
        shift-right: [w453] -> w421
        shift-left: FALSE -> [w452]
        tunnel: [w446] -> w420 mode=indexing
        n170 = Unbundle By Name(w450) -> ("String"=w446:string)
        n171 = call "Namen aus Tabelle ersetzen.vi"("Regulärer Ausdruck"=w446, "Sprachauswahl"=w447, "Tabelle"=w455) -> ("Übersetzung"=w449:string)  [unwired: 8 in]
        n172 = Empty String/Path?(string/path=w449) -> (empty?=w454:bool)
        n173 = Bundle By Name(cluster=w450, "String"=w449) -> (w448:cluster{"String":string, "Value":ext})
        n174 = Select(t=TRUE, s=w454, f=w452) -> (s? t:f=w453:bool)
      }
      n175 = case shown="False" w421 {
        tunnel: w428 -> [w443 w444]
        tunnel: w427 -> [w442 w445]
        tunnel: w423 -> [w441 _]
        tunnel: [w440 w444] -> w426
        tunnel: [w439 w445] -> w425
        frame False {
          n176 = property class="Ring"(reference=w442, error in=w443, "StringsAndValues[]"=w441) -> (reference out=w439:refnum<vi>, error out=w440:errorcluster)
        }
        frame True {
        }
      }
      n177 = Close Reference(reference=w425, error in (no error)=w426) -> (error out=w424:errorcluster)
      n178 = call <vilib>:"Clear Errors.vi"("error in (no error)"=w424) -> ("error out"=w419:errorcluster)  [unwired: 5 in, 1 out]
    }
    frame 46 {
      w477 = refnum<vi> refnum  # MehrspaltigesListenfeld
      w480 = refnum<vi> refnum  # Allgemein
      # "Eventuell die komplette Casestruktur mit allen funktionen einbauen?!!"
      n179 = To More Generic Class(target class=w480, reference=w481) -> (generic class reference=w479:refnum<vi>)
      n180 = To More Specific Class(target class=w477, reference=w479, error in=w478) -> (specific class reference=w471:refnum<vi>, error out=w476:errorcluster)
      n181 = property class="MehrSpaltFeld"(reference=w471, error in=w476) -> (reference out=w473:refnum<vi>, error out=w472:errorcluster, "RowHdrs[]"=w459:string[])
      n182 = property class="MehrSpaltFeld"(reference=w471) -> (reference out=w468:refnum<vi>, error out=w467:errorcluster, "ColHdrString"=w458:string[])  [unwired: 1 in]
      n183 = Build Array (concatenate)(w459, w458) -> (w457:string[])
      n184 = for {
        tunnel: w470 -> [w493]
        tunnel: w469 -> [w492]
        tunnel: w459 -> [w490] mode=indexing
        tunnel: [w488] -> w474 mode=indexing
        n185 = call "Namen aus Tabelle ersetzen.vi"("Regulärer Ausdruck"=w490, "Sprachauswahl"=w492, "Tabelle"=w493) -> ("Übersetzung"=w489:string)  [unwired: 8 in]
        n186 = Empty String/Path?(string/path=w489) -> (empty?=w491:bool)
        n187 = Select(t=w490, s=w491, f=w489) -> (s? t:f=w488:string)
      }
      n188 = for {
        tunnel: w470 -> [w487]
        tunnel: w469 -> [w486]
        tunnel: w458 -> [w482] mode=indexing
        tunnel: [w483] -> w466 mode=indexing
        n189 = call "Namen aus Tabelle ersetzen.vi"("Regulärer Ausdruck"=w482, "Sprachauswahl"=w486, "Tabelle"=w487) -> ("Übersetzung"=w484:string)  [unwired: 8 in]
        n190 = Empty String/Path?(string/path=w484) -> (empty?=w485:bool)
        n191 = Select(t=w482, s=w485, f=w484) -> (s? t:f=w483:string)
      }
      n192 = property class="MehrSpaltFeld"(reference=w468, error in=w467, "ColHdrString"=w466) -> (reference out=w461:refnum<vi>, error out=w463:errorcluster)
      n193 = property class="MehrSpaltFeld"(reference=w473, error in=w472, "RowHdrs[]"=w474) -> (reference out=w460:refnum<vi>, error out=w464:errorcluster)
      n194 = Merge Errors(w464, w463) -> (w462:errorcluster)
      n195 = Close Reference(reference=w460, error in (no error)=w462) -> (error out=w465:errorcluster)
      n196 = Close Reference(reference=w461, error in (no error)=w462) -> (error out=w475:errorcluster)
      n197 = call <vilib>:"Clear Errors.vi"("error in (no error)"=w465) -> ("error out"=w456:errorcluster)  [unwired: 5 in, 1 out]
      n198 = call <vilib>:"Clear Errors.vi"("error in (no error)"=w475) -> ()  [unwired: 5 in, 2 out]
    }
    frame 55 {
      w505 = refnum<vi> refnum  # Registerkartenelement
      w508 = refnum<vi> refnum  # Allgemein
      # "mit RKUntertitel schon - riw 11.07.2018 #BugFixSpracheRegisterkarten"
      # "Funktioniert nicht!!"
      n199 = To More Generic Class(target class=w508, reference=w509) -> (generic class reference=w507:refnum<vi>)
      n200 = To More Specific Class(target class=w505, reference=w507, error in=w506) -> (specific class reference=w504:refnum<vi>, error out=w503:errorcluster)
      n201 = property class="RKElem"(reference=w504, error in=w503) -> (error out=w502:errorcluster, "Pages"=w496:refnum<vi>[])  [unwired: 1 out]
      n202 = call "Registerkartenverwaltung.vi"("Sprachauswahl"=w495, "all rows"=w494, "Seiten"=w496) -> ()  [unwired: 9 in]
      n203 = for {
        tunnel: w502 -> [w520]
        tunnel: w496 -> [w519] mode=indexing
        tunnel: w495 -> [w513]
        tunnel: w494 -> [w518]
        tunnel: [w515] -> w501
        tunnel: [w514] -> w500
        tunnel: [w512] -> w498 mode=indexing
        n204 = property class="Seite"(reference=w519, error in=w520) -> (reference out=w511:refnum<vi>, error out=w517:errorcluster, "TabCaption"=w512:string)
        n205 = call "Namen aus Tabelle ersetzen.vi"("Regulärer Ausdruck"=w512, "Sprachauswahl"=w513, "Tabelle"=w518) -> ("Übersetzung"=w516:string)  [unwired: 8 in]
        n206 = Empty String/Path?(string/path=w516) -> (empty?=w510:bool)
        n207 = case shown="False" w510 {
          tunnel: w517 -> [w523 w527]
          tunnel: w511 -> [w526 w528]
          tunnel: [w524 w527] -> w514
          tunnel: [w525 w528] -> w515
          tunnel: w516 -> [w522 _]
          frame False {
            # "#BugFixSpracheRegisterkarten"
            n208 = property class="Seite"(reference=w526, error in=w523, "IndependentLabel"=TRUE ("Unabhängige Beschriftung"), "TabCaption"=w522) -> (reference out=w525:refnum<vi>, error out=w524:errorcluster)
          }
          frame True {
          }
        }
      }
      n209 = Close Reference(reference=w501, error in (no error)=w500) -> (error out=w499:errorcluster)
      n210 = call <vilib>:"Clear Errors.vi"("error in (no error)"=w499) -> ("error out"=w497:errorcluster)  [unwired: 5 in, 1 out]
    }
    frame 83 {
      w548 = refnum<vi> refnum  # XYGraph
      w551 = refnum<vi> refnum  # Allgemein
      n211 = To More Generic Class(target class=w551, reference=w552) -> (generic class reference=w550:refnum<vi>)
      n212 = To More Specific Class(target class=w548, reference=w550, error in=w549) -> (specific class reference=w547:refnum<vi>, error out=w546:errorcluster)
      n213 = property class="XYGraph"(reference=w547, error in=w546) -> (reference out=w542:refnum<vi>, error out=w540:errorcluster, "XScale.NameLbl.Text"=w545:string, "YScale.NameLbl.Text"=w544:string)
      n214 = Build Array(w545, w544) -> (w532:string[])
      n215 = for {
        N: 10 -> [_]
        tunnel: w542 -> [w566]
        tunnel: w540 -> [w562]
        tunnel: w537 -> [w561]
        tunnel: w536 -> [w560]
        tunnel: [w555] -> w534
        tunnel: [w554] -> w533
        tunnel: [w553] -> w531 mode=indexing
        i -> [w565]
        n216 = property class="XYGraph"(reference=w566, error in=w562, "Active Plot"=w565) -> (reference out=w564:refnum<vi>, error out=w563:errorcluster)
        n217 = property class="XYGraph"(reference=w564, error in=w563) -> (reference out=w558:refnum<vi>, error out=w557:errorcluster, "Plot.Plot Name"=w559:string)
        n218 = call "Namen aus Tabelle ersetzen.vi"("Regulärer Ausdruck"=w559, "Sprachauswahl"=w560, "Tabelle"=w561) -> ("Übersetzung"=w553:string)  [unwired: 8 in]
        n219 = Empty String/Path?(string/path=w553) -> (empty?=w556:bool)
        n220 = case shown="True" w556 {
          tunnel: w558 -> [w571 w573]
          tunnel: w557 -> [w570 w572]
          tunnel: [w569 w573] -> w555
          tunnel: [w568 w572] -> w554
          tunnel: w553 -> [w567 _]
          frame False {
            n221 = property class="XYGraph"(reference=w571, error in=w570, "Plot.Plot Name"=w567) -> (reference out=w569:refnum<vi>, error out=w568:errorcluster)
          }
          frame True {
          }
        }
      }
      n222 = for {
        tunnel: w537 -> [w584]
        tunnel: w536 -> [w575]
        tunnel: w532 -> [w574] mode=indexing
        tunnel: w542 -> [w579]
        tunnel: w540 -> [w578]
        tunnel: [w577] -> w539
        tunnel: [w576] -> w538
        i -> [w581]
        n223 = Not Equal To 0?(x=w581) -> (x != 0?=w580:bool)
        n224 = call "Namen aus Tabelle ersetzen.vi"("Regulärer Ausdruck"=w574, "Sprachauswahl"=w575, "Tabelle"=w584) -> ("Übersetzung"=w582:string)  [unwired: 8 in]
        n225 = Empty String/Path?(string/path=w582) -> (empty?=w583:bool)
        n226 = case shown="True" w580 {
          tunnel: w583 -> [w590 w603]
          tunnel: w582 -> [w589 w602]
          tunnel: w579 -> [w588 w601]
          tunnel: w578 -> [w587 w600]
          tunnel: [w586 w598] -> w576
          tunnel: [w585 w599] -> w577
          frame True {
            n227 = case shown="True" w590 {
              tunnel: w587 -> [w595 w596]
              tunnel: w588 -> [w594 w597]
              tunnel: [w593 w596] -> w586
              tunnel: [w592 w597] -> w585
              tunnel: w589 -> [w591 _]
              frame False {
                n228 = property class="XYGraph"(reference=w594, error in=w595, "YScale.NameLbl.Text"=w591) -> (reference out=w592:refnum<vi>, error out=w593:errorcluster)
              }
              frame True {
              }
            }
          }
          frame False {
            n229 = case shown="True" w603 {
              tunnel: w600 -> [w608 w609]
              tunnel: w601 -> [w607 w610]
              tunnel: [w606 w609] -> w598
              tunnel: [w605 w610] -> w599
              tunnel: w602 -> [w604 _]
              frame False {
                n230 = property class="XYGraph"(reference=w607, error in=w608, "XScale.NameLbl.Text"=w604) -> (reference out=w605:refnum<vi>, error out=w606:errorcluster)
              }
              frame True {
              }
            }
          }
        }
      }
      n231 = Close Reference(reference=w534, error in (no error)=w533) -> (error out=w535:errorcluster)
      n232 = Close Reference(reference=w539, error in (no error)=w538) -> (error out=w543:errorcluster)
      n233 = Build Array (concatenate)(w532, w531) -> (w530:string[])
      n234 = call <vilib>:"Clear Errors.vi"("error in (no error)"=w535) -> ()  [unwired: 5 in, 2 out]
      n235 = call <vilib>:"Clear Errors.vi"("error in (no error)"=w543) -> ("error out"=w529:errorcluster)  [unwired: 5 in, 1 out]
    }
  }
  "Strings [4]" <- w12
  "Cluster Elemente[]" <- w7
  "error out" <- w6
